vi "initialize_data_log.vi"(7 "Overwrite?":bool, 8 "error in (no error)":errorcluster, 9 "Initialization Data":variant, 10 "Path":path, 11 "tt20_logger in":refnum<class "tt20_logger.lvclass">) -> (0 "error out":errorcluster, 3 "tt20_logger out":refnum<class "tt20_logger.lvclass">)   [LabVIEW 2015, in "tt20_logger.lvclass"]
uses:
  tt20_logger.lvclass
  tt20_logger.lvclass/tt20_logger.ctl
  <vilib>/UPVI/lvhdf5/file.llb/LVH5F Operation.ctl
  <vilib>/UPVI/lvhdf5/property.llb/LVH5PClassId.ctl
  <vilib>/UPVI/lvhdf5/dataset.llb/LVH5D Operation.ctl
  <vilib>/UPVI/lvhdf5/datatype.llb/LVH5Tcreate_dataset_type (Variant).vi
  <vilib>/UPVI/lvhdf5/datatype.llb/LVH5Tcreate_dataset_type.xnode
  <vilib>/UPVI/lvhdf5/library.llb/HDF5 Ref.ctl
  Picoquant/Hydraharp/hydraharp/hydraharp.lvclass
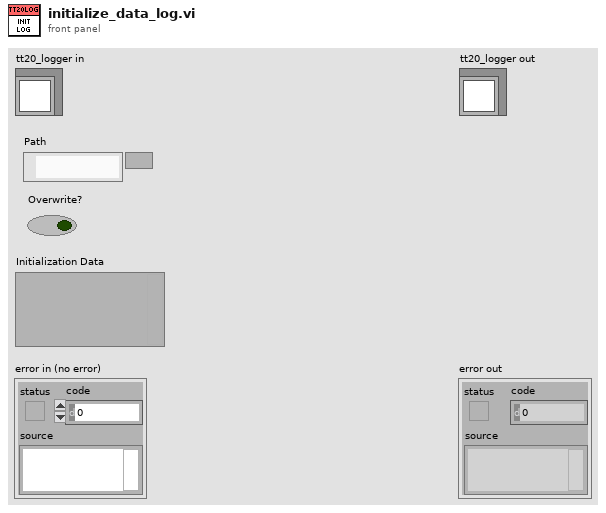
[diagram p1: front panel]
types:
  T1 = typedef "LVH5F Operation.ctl" = enum16{"open", "open or create", "create or replace", "create or replace (with confirmation)", "create", "open (read only)"}
  T2 = typedef "HDF5 Ref.ctl" = refnum<k1>
  T3 = typedef "LVH5D Operation.ctl" = enum16{"open", "replace", "create", "open or create", "create or replace", "create or replace with confirmation"}
  T4 = typedef "LVH5PClassId.ctl" = enum32{"H5P_ROOT", "H5P_OBJECT_CREATE", "H5P_FILE_CREATE", "H5P_FILE_ACCESS", "H5P_DATASET_CREATE", "H5P_DATASET_ACCESS", "H5P_DATASET_XFER", "H5P_FILE_MOUNT", "H5P_GROUP_CREATE", "H5P_GROUP_ACCESS", "H5P_DATATYPE_CREATE", "H5P_DATATYPE_ACCESS", "H5P_STRING_CREATE", "H5P_ATTRIBUTE_CREATE", "H5P_OBJECT_COPY", "H5P_LINK_CREATE", "H5P_LINK_ACCESS"}
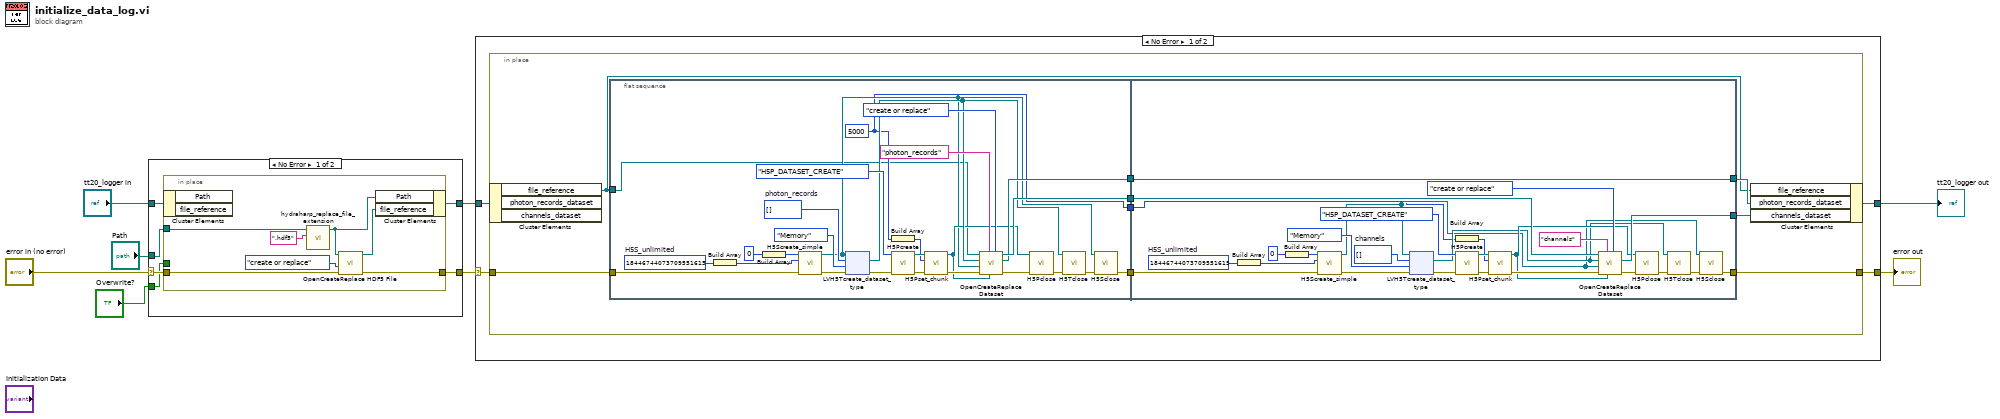
[diagram p0: block diagram]
diagram:
  n1 = case shown="No Error" "error in (no error)" {
    selector: "error in (no error)" -> [w13 w23]
    tunnel: "tt20_logger in" -> [w14 w22]
    tunnel: "Path" -> [w12 _]
    tunnel: "Overwrite?" -> [w11 _]
    tunnel: [w10 w22] -> w4
    tunnel: [w9 w23] -> w3
    frame No Error {
      n2 = in-place {
        in-place-border: w13 -> [w21]
        in-place-border: w12 -> [w20]
        in-place-border: w11 -> [_]
        in-place-border: [w16] -> w9
        n3 = in-place-cluster #1(w14) -> ()  [unwired: 2 out]
        n4 = call "hydraharp_replace_file_extension.vi"("new_extension"=".hdf5", "input_file"=w20) -> ("new_name"=w17:path)  [unwired: 9 in]
        n5 = call <vilib>:"OpenCreateReplace HDF5 File.vi"("error in (no error)"=w21, "function (open or create)"=LVH5F_Operation."create or replace", "path"=w17) -> ("error out"=w16:errorcluster, "HDF5 Ref out"=w18:T2)  [unwired: 5 in]
        n6 = in-place-cluster #1("Path"=w17, "file_reference"=w18) -> (w10:refnum<class "tt20_logger.lvclass">)
      }
    }
    frame Error {
    }
  }
  n7 = case shown="No Error" w3 {
    selector: w3 -> [w27 w140]
    tunnel: [w26 w139] -> w2
    tunnel: [w25 w140] -> w1
    tunnel: w4 -> [w24 w139]
    frame No Error {
      n8 = in-place {
        in-place-border: w27 -> [w29]
        in-place-border: [w30] -> w25
        n9 = in-place-cluster #2(w24) -> ("file_reference"=w28:T2)  [unwired: 2 out]
        n10 = flat-sequence {
          tunnel: [w50] -> w35
          tunnel: [w48] -> w34
          tunnel: [w43] -> w32
          tunnel: [w39] -> w31
          tunnel: w28 -> [w38]
          tunnel: w29 -> [w37]
          tunnel: w35 -> [w102]
          tunnel: w34 -> [w114]
          tunnel: [w101] -> w33
          tunnel: w32 -> [w103]
          tunnel: w31 -> [w93]
          tunnel: [w114] -> w36
          tunnel: [w88] -> w30
          frame #0 {
            w39 = 5000
            w54 = u64[] []  # photon_records
            w58 = u64 18446744073709551615  # H5S_unlimited
            n11 = Build Array(w58) -> (w57:u64[])
            n12 = Build Array(u64 0 ("element")) -> (w55:u64[])
            n13 = call <vilib>:"H5Screate_simple.vi"("error in (no error)"=w37, "Maximum Dimensions (unlimited)"=w57, "Dimensions"=w55) -> ("error out"=w63:errorcluster, "HDF5 Ref out"=w40:T2)  [unwired: 5 in]
            n14 = xnode "LVH5Tcreate_dataset_type"("HDF5 Location Ref"=w40, "Type"=enum16{"File", "Memory"}."Memory", "error in (no error)"=w63, "Data"=w54) -> ("HDF5 Type Ref"=w42:T2, "error out"=w60:errorcluster)  [unwired: 2 in, 3 out]
            n15 = Build Array(w39) -> (w51:i32[])
            n16 = call <vilib>:"H5Pcreate.vi"("error in (no error)"=w60, "Property List Class"=LVH5PClassId."H5P_DATASET_CREATE") -> ("error out"=w61:errorcluster, "HDF5 Property List Ref"=w62:T2)  [unwired: 6 in]
            n17 = call <vilib>:"H5Pset_chunk.vi"("error in (no error)"=w61, "Dimensions"=w51, "HDF5 Property Ref"=w62) -> ("error out"=w59:errorcluster, "HDF5 Ref out"=w41:T2)  [unwired: 5 in]
            n18 = call <vilib>:"OpenCreateReplace Dataset.vi"("operation (open or create)"=LVH5D_Operation."create or replace", "HDF5 Property List Ref"=w41, "Dataset Path"="photon_records" ("string"), "error in (no error)"=w59, "HDF5 Dataspace Ref"=w40, "HDF5 Datatype Ref"=w42, "HDF5 Ref"=w38) -> ("error out"=w44:errorcluster, "HDF5 Dataset Ref"=w48:T2, "HDF5 Ref out"=w50:T2)  [unwired: 2 in]
            n19 = call <vilib>:"H5Pclose.vi"("error in (no error)"=w44, "HDF5 Property Ref"=w41) -> ("error out"=w46:errorcluster)  [unwired: 7 in]
            n20 = call <vilib>:"H5Tclose.vi"("error in (no error)"=w46, "HDF5 Datatype Ref"=w42) -> ("error out"=w45:errorcluster)  [unwired: 7 in]
            n21 = call <vilib>:"H5Sclose.vi"("error in (no error)"=w45, "HDF5 Dataspace Ref"=w40) -> ("error out"=w43:errorcluster)  [unwired: 7 in]
          }
          frame #1 {
            w92 = u64 18446744073709551615  # H5S_unlimited
            w108 = u8[] []  # channels
            n22 = Build Array(w92) -> (w90:u64[])
            n23 = Build Array(u64 0 ("element")) -> (w89:u64[])
            n24 = call <vilib>:"H5Screate_simple.vi"("error in (no error)"=w103, "Maximum Dimensions (unlimited)"=w90, "Dimensions"=w89) -> ("error out"=w113:errorcluster, "HDF5 Ref out"=w94:T2)  [unwired: 5 in]
            n25 = xnode "LVH5Tcreate_dataset_type"("HDF5 Location Ref"=w94, "Type"=enum16{"File", "Memory"}."Memory", "error in (no error)"=w113, "Data"=w108) -> ("HDF5 Type Ref"=w95:T2, "error out"=w110:errorcluster)  [unwired: 2 in, 3 out]
            n26 = Build Array(w93) -> (w105:i32[])
            n27 = call <vilib>:"H5Pcreate.vi"("error in (no error)"=w110, "Property List Class"=LVH5PClassId."H5P_DATASET_CREATE") -> ("error out"=w111:errorcluster, "HDF5 Property List Ref"=w112:T2)  [unwired: 6 in]
            n28 = call <vilib>:"H5Pset_chunk.vi"("error in (no error)"=w111, "Dimensions"=w105, "HDF5 Property Ref"=w112) -> ("error out"=w109:errorcluster, "HDF5 Ref out"=w96:T2)  [unwired: 5 in]
            n29 = call <vilib>:"OpenCreateReplace Dataset.vi"("operation (open or create)"=LVH5D_Operation."create or replace", "HDF5 Property List Ref"=w96, "Dataset Path"="channels" ("string"), "error in (no error)"=w109, "HDF5 Dataspace Ref"=w94, "HDF5 Datatype Ref"=w95, "HDF5 Ref"=w102) -> ("error out"=w97:errorcluster, "HDF5 Dataset Ref"=w101:T2)  [unwired: 2 in, 1 out]
            n30 = call <vilib>:"H5Pclose.vi"("error in (no error)"=w97, "HDF5 Property Ref"=w96) -> ("error out"=w99:errorcluster)  [unwired: 7 in]
            n31 = call <vilib>:"H5Tclose.vi"("error in (no error)"=w99, "HDF5 Datatype Ref"=w95) -> ("error out"=w98:errorcluster)  [unwired: 7 in]
            n32 = call <vilib>:"H5Sclose.vi"("error in (no error)"=w98, "HDF5 Dataspace Ref"=w94) -> ("error out"=w88:errorcluster)  [unwired: 7 in]
          }
        }
        n33 = in-place-cluster #2("file_reference"=w28, "photon_records_dataset"=w36, "channels_dataset"=w33) -> (w26:refnum<class "tt20_logger.lvclass">)
      }
    }
    frame Error {
    }
  }
  "error out" <- w1
  "tt20_logger out" <- w2
